vi "pub_multipart.vi"() -> ()   [LabVIEW 2010]
uses:
  socket_type.ctl
  zeromq.lvlib
  zmq_context.lvclass
  zmq_socket.lvclass
panel:
  out "message":string[](array[string])
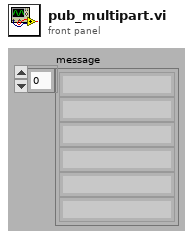
[diagram p1: front panel]
types:
  T1 = typedef "zeromq.lvlib/socket_type.ctl" = enum8{"ZMQ_PAIR", "ZMQ_PUB", "ZMQ_SUB", "ZMQ_REQ", "ZMQ_REP", "ZMQ_DEALER", "ZMQ_ROUTER", "ZMQ_PULL", "ZMQ_PUSH", "ZMQ_XPUB", "ZMQ_XSUB"}
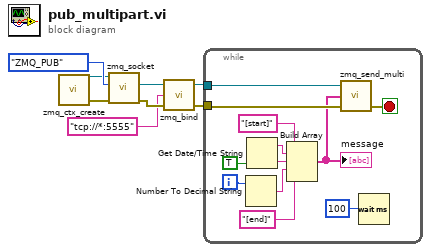
[diagram p0: block diagram]
diagram:
  n1 = call "zmq_ctx_create.vi"() -> ("error out"=w6:errorcluster, "context out"=w3:refnum<class "zmq_context.lvclass">)  [unwired: 4 in]
  n2 = call "zmq_socket.vi"("error in"=w6, "socket type"=socket_type."ZMQ_PUB", "context in"=w3) -> ("error out"=w5:errorcluster, "socket out"=w2:refnum<class "zmq_socket.lvclass">)  [unwired: 2 in, 1 out]
  n3 = call "zmq_bind.vi"("error in"=w5, "endpoint"="tcp://*:5555", "socket in"=w2) -> ("error out"=w4:errorcluster, "socket out"=w8:refnum<class "zmq_socket.lvclass">)  [unwired: 1 in]
  n4 = while {
    tunnel: w8 -> [w19]
    tunnel: w4 -> [w18]
    i -> [w9]
    stop <- w17 stop-if-true
    n5 = Number To Decimal String(number=w9) -> (decimal integer string=w11:string)  [unwired: 1 in]
    n6 = Get Date/Time String(want seconds? (F)=TRUE) -> (date string=w16:string, time string=w15:string)  [unwired: 2 in]
    n7 = Build Array("[start]" ("element"), w16, w15, w11, "[end]" ("element")) -> (w13:string[])
    "message" <- w13
    n8 = call "zmq_send_multi.vi"("error in"=w18, "parts"=w13, "socket in"=w19) -> ("error out"=w17:errorcluster)  [unwired: 1 in, 1 out]
    n9 = Wait (ms)(milliseconds to wait=u32 100) -> ()  [unwired: 1 out]
  }
